vi "init ZeroMQ VIs.vi"(8 "error in (no error)":errorcluster, 11 "Header content in":refnum<class "Header content.lvclass">) -> (0 "error out":errorcluster, 3 "Header content out":refnum<class "Header content.lvclass">)   [LabVIEW 2018, in "Header content.lvclass"]
uses:
  Header content.lvclass
  Header content.lvclass/Header content.ctl
  Server/Server.lvclass/Server.ctl
  Server/Server.lvclass
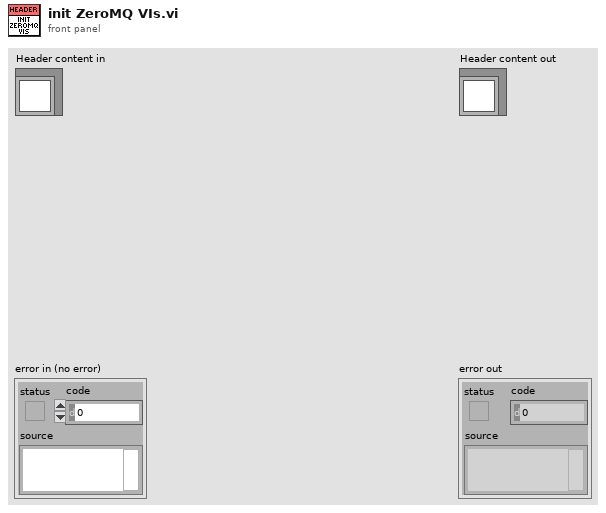
[diagram p1: front panel]
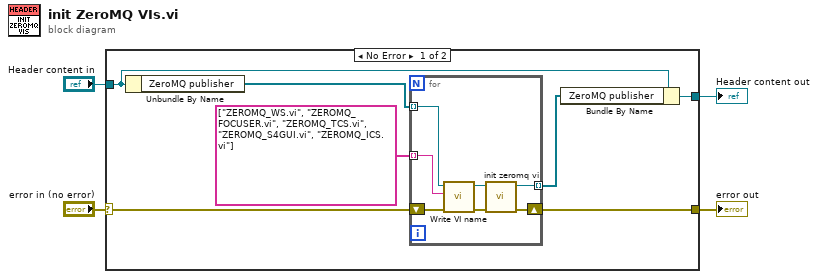
[diagram p0: block diagram]
diagram:
  n1 = case shown="No Error" "error in (no error)" {
    selector: "error in (no error)" -> [w10 w20]
    tunnel: [w9 w20] -> w3
    tunnel: [w8 w19] -> w1
    tunnel: "Header content in" -> [w7 w19]
    frame No Error {
      n2 = Unbundle By Name(w7) -> ("ZeroMQ publisher"=w6:refnum<class "Server.lvclass">[])
      n3 = for {
        tunnel: string[] ["ZEROMQ_WS.vi", "ZEROMQ_FOCUSER.vi", "ZEROMQ_TCS.vi", "ZEROMQ_S4GUI.vi", "ZEROMQ_ICS.vi"] -> [w14] mode=indexing
        shift-right: [w13] -> w9
        shift-left: w10 -> [w16]
        tunnel: w6 -> [w15] mode=indexing
        tunnel: [w12] -> w5 mode=indexing
        n4 = call "Write VI name.vi"("error in (no error)"=w16, "VI name"=w14, "Server in"=w15) -> ("error out"=w17:errorcluster, "Server out"=w18:refnum<class "Server.lvclass">)  [unwired: 7 in]
        n5 = call "init zeromq vi.vi"("error in (no error)"=w17, "Server in"=w18) -> ("error out"=w13:errorcluster, "Server out"=w12:refnum<class "Server.lvclass">)  [unwired: 8 in]
      }
      n6 = Bundle By Name(cluster=w7, "ZeroMQ publisher"=w5) -> (w8:refnum<class "Header content.lvclass">)
    }
    frame Error {
    }
  }
  "error out" <- w3
  "Header content out" <- w1
